vi "task4.vi"() -> ()   [LabVIEW 2021]
uses:
  <vilib>/Utility/file.llb/Write Delimited Spreadsheet (DBL).vi
panel:
  out "Waveform Graph":dbl[](graph)
  in  "file path (dialog if empty)":path
  in  "sampling time":u32
  in  "Samples":i32
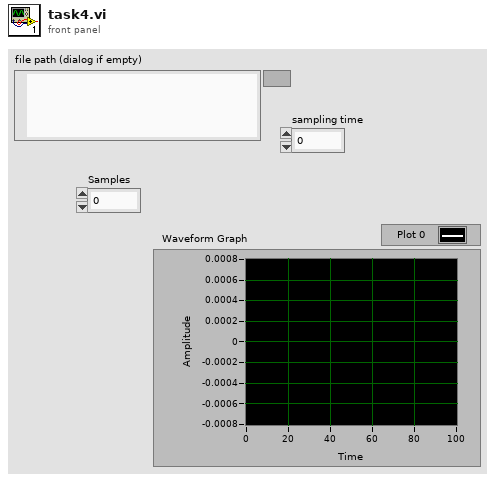
[diagram p1: front panel]
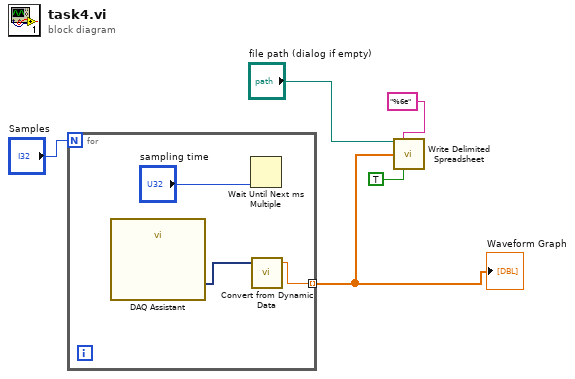
[diagram p0: block diagram]
diagram:
  n1 = for {
    N: "Samples" -> [_]
    tunnel: [w6] -> w1 mode=indexing
    n2 = call "DAQ Assistant"() -> ("data"=w7:dynamicdata)  [unwired: 17 in, 2 out]
    n3 = Wait Until Next ms Multiple(millisecond multiple="sampling time") -> ()  [unwired: 1 out]
    n4 = call "Convert from Dynamic Data"("Dynamic Data Type"=w7) -> ("Scalar"=w6:dbl)  [unwired: 3 in]
  }
  "Waveform Graph" <- w1
  n5 = call-poly <vilib>:"Write Delimited Spreadsheet.vi"("file path (dialog if empty)"="file path (dialog if empty)", "format (%.3f)"="%6e", "1D data"=w1, "transpose? (no:F)"=TRUE) -> ()  [unwired: 10 in, 2 out]
